vi "CT2.vi"(3 "Total time":dbl, 8 "dir info":cluster{"first dir":bool, "alternate dir":bool}={"first dir"=TRUE, "alternate dir"=FALSE}, 11 "mode":u16(ring)=1 items=["initial time", "count time", "reset time"]) -> (0 "time end ?":bool, 1 "variate time":dbl, 2 "output count time":T1)   [LabVIEW 2011]
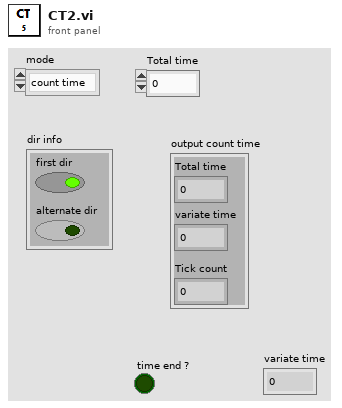
[diagram p1: front panel]
types:
  T1 = cluster{"Total time":dbl, "variate time":dbl, "Tick count":u32}
  T2 = cluster{"Total time":dbl, dbl, "millisecond timer value":u32}
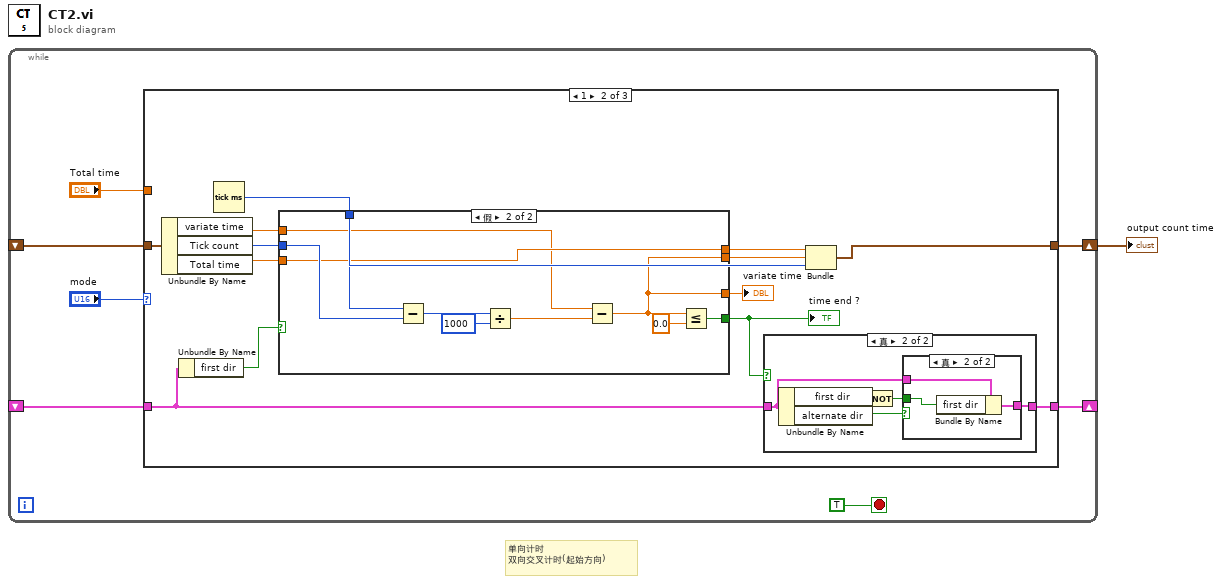
[diagram p0: block diagram]
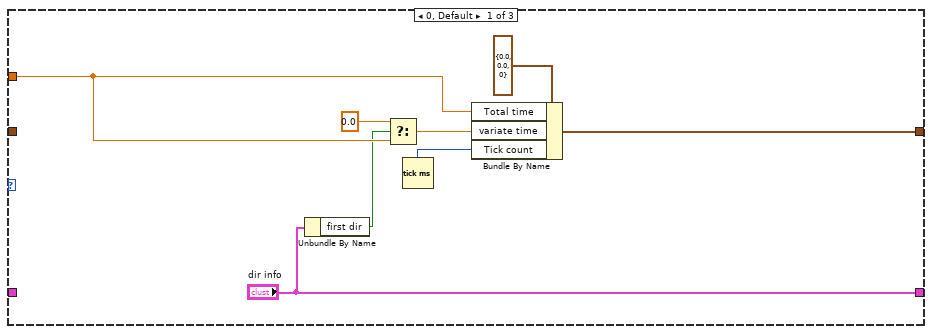
[diagram p2: hidden frame]
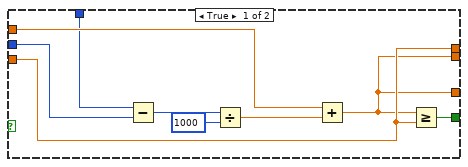
[diagram p5: hidden frame]
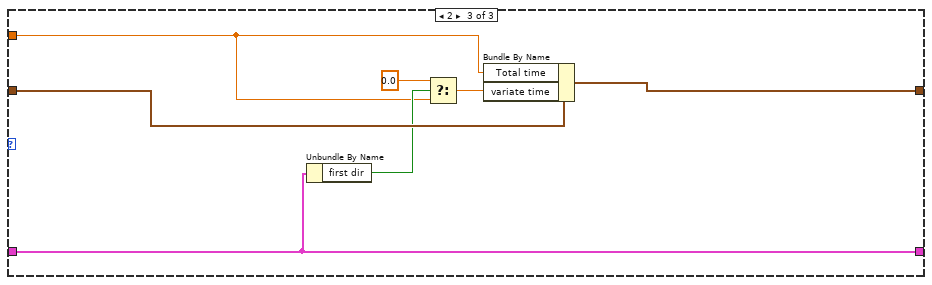
[diagram p6: hidden frame]
diagram:
  # "单向计时\n双向交叉计时(起始方向)"
  n1 = while {
    shift-right: [w7] -> w1
    shift-left: _ -> [w8]
    shift-right: [w3] -> _
    shift-left: _ -> [w2]
    stop <- TRUE stop-if-true
    n2 = case shown="1" "mode" {
      tunnel: w8 -> [_ w29 w65]
      tunnel: [w14 w24 w64] -> w7
      tunnel: "Total time" -> [w12 _ w60]
      tunnel: ["dir info" w17 w59] -> w3
      tunnel: w2 -> [_ w19 w59]
      frame 0, Default {
        n3 = Unbundle By Name("dir info") -> ("first dir"=w9:bool)
        n4 = Select(t=0.0, s=w9, f=w12) -> (s? t:f=w11:dbl)
        n5 = Tick Count (ms)() -> (millisecond timer value=w15:u32)
        n6 = Bundle By Name(cluster=T1 {"Total time"=0.0, "variate time"=0.0, "Tick count"=0} ("output count time 2"), "Total time"=w12, "variate time"=w11, "Tick count"=w15) -> (w14:T1)
      }
      frame 1 {
        n7 = Unbundle By Name(w29) -> ("variate time"=w27:dbl, "Tick count"=w28:u32, "Total time"=w23:dbl)
        n8 = Unbundle By Name(w19) -> ("first dir"=w20:bool)
        n9 = Tick Count (ms)() -> (millisecond timer value=w25:u32)
        n10 = case shown="假" w20 {
          tunnel: [w48 w58] -> w18
          tunnel: w28 -> [w44 w54]
          tunnel: w27 -> [w43 w49]
          tunnel: [w40 w52] -> w26
          tunnel: w25 -> [w42 w53]
          tunnel: w23 -> [w41 w50]
          tunnel: [w41 w50] -> w22
          tunnel: [w40 w52] -> w21
          frame True {
            n11 = Subtract(x=w42, y=w44) -> (x-y=w45:u32)
            n12 = Divide(x=w45, y=u32 1000) -> (x/y=w47:dbl)
            n13 = Add(x=w43, y=w47) -> (x+y=w40:dbl)
            n14 = Greater Or Equal?(x=w40, y=w41) -> (x >= y?=w48:bool)
          }
          frame False {
            n15 = Subtract(x=w53, y=w54) -> (x-y=w55:u32)
            n16 = Divide(x=w55, y=u32 1000) -> (x/y=w57:dbl)
            n17 = Subtract(x=w49, y=w57) -> (x-y=w52:dbl)
            n18 = Less Or Equal?(x=w52, y=0.0) -> (x <= y?=w58:bool)
          }
        }
        "time end ?" <- w18
        "variate time" <- w21
        n19 = case shown="真" w18 {
          tunnel: w19 -> [w30 w33]
          tunnel: [w30 w32] -> w17
          frame False {
          }
          frame True {
            n20 = Unbundle By Name(w33) -> ("first dir"=w34:bool, "alternate dir"=w35:bool)
            n21 = Not(x=w34) -> (.not. x?=w31:bool)
            n22 = case shown="真" w35 {
              tunnel: w33 -> [w36 w39]
              tunnel: [w36 w38] -> w32
              tunnel: w31 -> [_ w37]
              frame False {
              }
              frame True {
                n23 = Bundle By Name(cluster=w39, "first dir"=w37) -> (w38:cluster{"first dir":bool, "alternate dir":bool})
              }
            }
          }
        }
        n24 = Bundle("Total time"=w22, w26, "millisecond timer value"=w25) -> (w24:T2)  [unwired: 1 in]
      }
      frame 2 {
        n25 = Unbundle By Name(w59) -> ("first dir"=w62:bool)
        n26 = Select(t=0.0, s=w62, f=w60) -> (s? t:f=w61:dbl)
        n27 = Bundle By Name(cluster=w65, "Total time"=w60, "variate time"=w61) -> (w64:T1)
      }
    }
  }
  "output count time" <- w1
